vi "DOConfigure.vi"(0 "object in":refnum<class "AD2_DO_SDK.lvclass">, 5 "error in (no error)":errorcluster) -> (14 "object out":refnum<class "AD2_DO_SDK.lvclass">, 19 "error out":errorcluster)   [LabVIEW 2021, in "AD2_DO_SDK.lvclass"]
uses:
  AD2_DO_SDK.lvclass
  AD2_DO_SDK.lvclass/AD2_DO_SDK.ctl
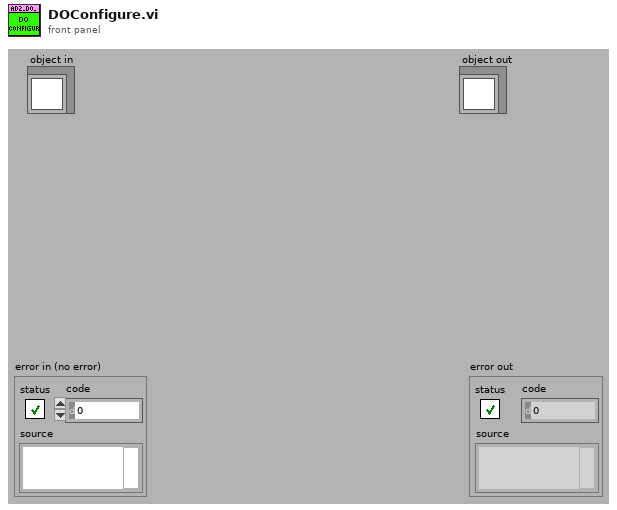
[diagram p1: front panel]
types:
  T1 = typedef "AD2_DO_SDK.lvclass/DOSingleCh.ctl" = cluster{"Ch Index":i32, "Enable":bool, "Clock DIvider":u32, "Type":i32, "DigitalOutOutput":u16, "IdleState":u16, "CounterData":cluster{"NoHighBits":u32, "NoLowBits":u32, "NoInitialBits":u32, "Start High":bool}, "Custom Data":cluster{"countOfBits":u32, "rgBits":u8[]}}
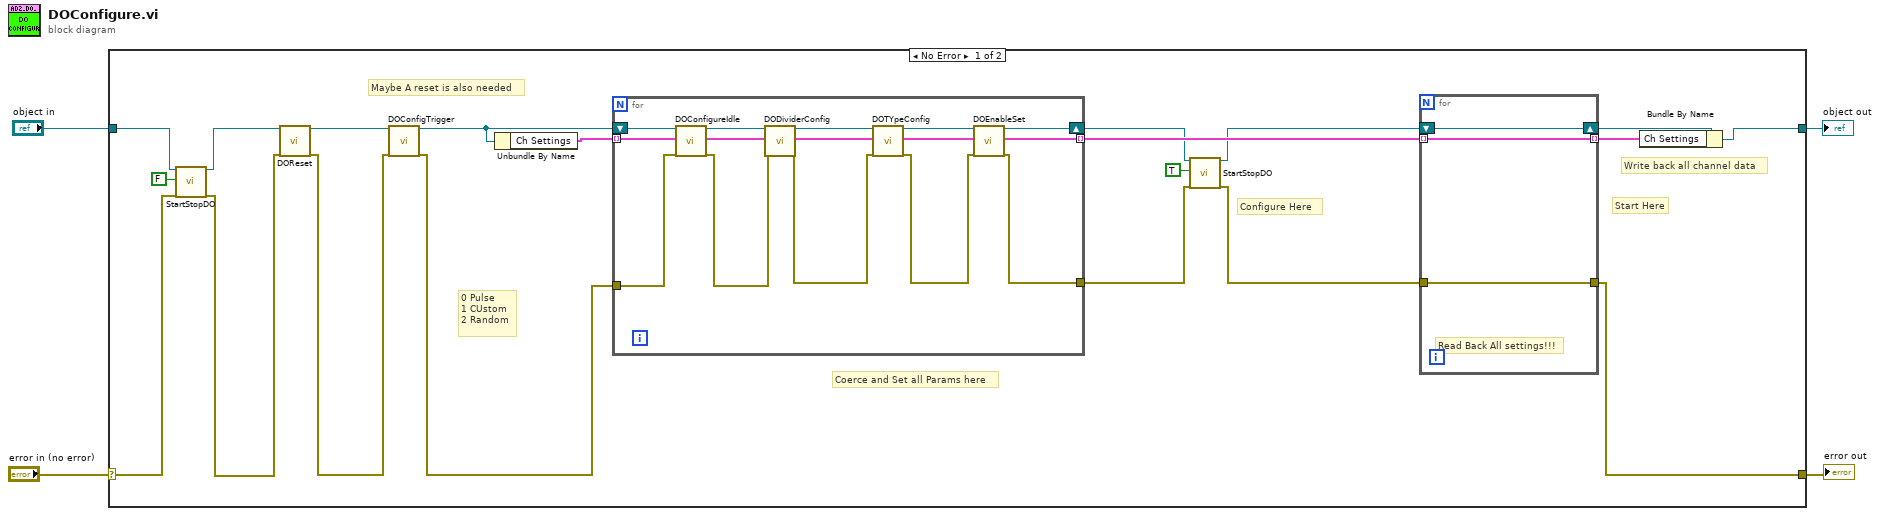
[diagram p0: block diagram]
diagram:
  n1 = case shown="No Error" "error in (no error)" {
    selector: "error in (no error)" -> [w6 w44]
    tunnel: [w19 w44] -> w3
    tunnel: [w23 w43] -> w1
    tunnel: "object in" -> [w7 w43]
    frame No Error {
      # "Maybe A reset is also needed"
      # "Start Here"
      # "Coerce and Set all Params here"
      # "Configure Here"
      # "Write back all channel data"
      # "0 Pulse\n1 CUstom\n2 Random"
      n2 = call-dynamic "StartStopDO.vi"("object in"=w7, "Running"=FALSE, "error in (no error)"=w6) -> ("object out"=w8:refnum<class "AD2_DO_SDK.lvclass">, "error out"=w5:errorcluster)  [unwired: 15 in]
      n3 = call-dynamic "DOReset.vi"("object in"=w8, "error in (no error)"=w5) -> ("object out"=w11:refnum<class "AD2_DO_SDK.lvclass">, "error out"=w10:errorcluster)  [unwired: 16 in]
      n4 = call-dynamic "DOConfigTrigger.vi"("object in"=w11, "error in (no error)"=w10) -> ("object out"=w13:refnum<class "AD2_DO_SDK.lvclass">, "error out"=w12:errorcluster)  [unwired: 16 in]
      n5 = Unbundle By Name(w13) -> ("Ch Settings"=w24:T1[])
      n6 = for {
        tunnel: w24 -> [w30] mode=indexing
        shift-right: [w36] -> w18
        shift-left: w13 -> [w33]
        tunnel: [w38] -> w22 mode=indexing
        tunnel: w12 -> [w28]
        tunnel: [w34] -> w16
        n7 = call-dynamic "DOConfigureIdle.vi"("object in"=w33, "DOSingleCh"=w30, "error in (no error)"=w28) -> ("object out"=w32:refnum<class "AD2_DO_SDK.lvclass">, "DOSingleCh"=w31:T1, "error out"=w29:errorcluster)  [unwired: 14 in]
        n8 = call-dynamic "DODividerConfig.vi"("object in"=w32, "DOSingleCh"=w31, "error in (no error)"=w29) -> ("object out"=w41:refnum<class "AD2_DO_SDK.lvclass">, "DOSingleCh Out"=w42:T1, "error out"=w40:errorcluster)  [unwired: 14 in]
        n9 = call-dynamic "DOTYpeConfig.vi"("object in"=w41, "DOSingleCh"=w42, "error in (no error)"=w40) -> ("object out"=w37:refnum<class "AD2_DO_SDK.lvclass">, "DOSingleCh Out"=w39:T1, "error out"=w35:errorcluster)  [unwired: 14 in]
        n10 = call-dynamic "DOEnableSet.vi"("object in"=w37, "DOSingleCh"=w39, "error in (no error)"=w35) -> ("object out"=w36:refnum<class "AD2_DO_SDK.lvclass">, "DOSingleCh Out"=w38:T1, "error out"=w34:errorcluster)  [unwired: 14 in]
      }
      n11 = call-dynamic "StartStopDO.vi"("object in"=w18, "Running"=TRUE, "error in (no error)"=w16) -> ("object out"=w17:refnum<class "AD2_DO_SDK.lvclass">, "error out"=w15:errorcluster)  [unwired: 15 in]
      n12 = for {
        tunnel: w22 -> [w27] mode=indexing
        tunnel: [w27] -> w21 mode=indexing
        shift-right: [w26] -> w20
        shift-left: w17 -> [w26]
        tunnel: [w25] -> w19
        tunnel: w15 -> [w25]
        # "Read Back All settings!!!"
      }
      n13 = Bundle By Name(cluster=w20, "Ch Settings"=w21) -> (w23:refnum<class "AD2_DO_SDK.lvclass">)
    }
    frame Error {
    }
  }
  "error out" <- w3
  "object out" <- w1
